vi "Turn off heating pins (SILAR).vi"(0 "Arduino Resource In":T1={"VISA resource"="", "Board Type"=enum."Uno", "Connection Type"=enum."USB / Serial", "Bytes Per Packet (15)"=15}, 5 "Error In":errorcluster) -> (14 "Arduino Resource Out":T1={"VISA resource"="", "Board Type"=enum."Uno", "Connection Type"=enum."USB / Serial", "Bytes Per Packet (15)"=15}, 19 "Error Out":errorcluster)   [LabVIEW 2012]
uses:
  <vilib>/LabVIEW Interface for Arduino/Type Defs/Arduino Resource.ctl
  <vilib>/LabVIEW Interface for Arduino/Type Defs/Board Type.ctl
  <vilib>/LabVIEW Interface for Arduino/LabVIEW Interface for Arduino.lvlib
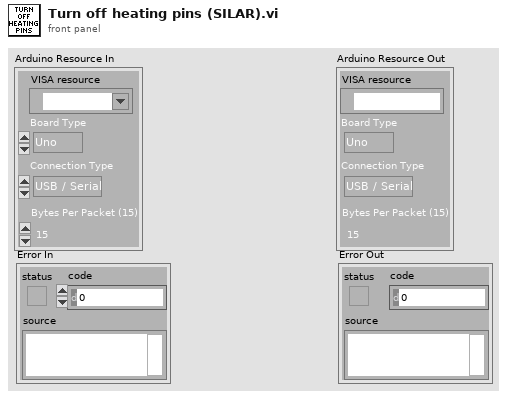
[diagram p1: front panel]
types:
  T1 = typedef "LabVIEW Interface for Arduino.lvlib/Arduino Resource.ctl" = cluster{"VISA resource":refnum<visa-resource-name>, "Board Type":T2, "Connection Type":enum8{"USB / Serial"}, "Bytes Per Packet (15)":u8}
  T2 = typedef "LabVIEW Interface for Arduino.lvlib/Board Type.ctl" = enum16{"Uno", "Dimuelanove w/Atmega 328", "Mega 2560"}
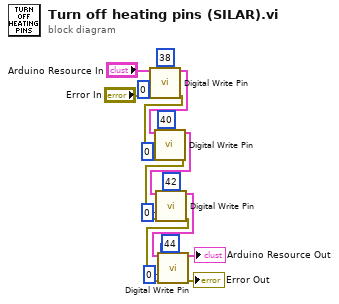
[diagram p0: block diagram]
diagram:
  n1 = call <vilib>:"Digital Write Pin.vi"("Arduino Resource"="Arduino Resource In", "Digital I/O Pin (0)"=u8 38, "Value (0)"=u8 0, "error in"="Error In") -> ("Arduino Resource"=w15:T1, "error out"=w16:errorcluster)  [unwired: 10 in]
  n2 = call <vilib>:"Digital Write Pin.vi"("Arduino Resource"=w15, "Digital I/O Pin (0)"=u8 40, "Value (0)"=u8 0, "error in"=w16) -> ("Arduino Resource"=w9:T1, "error out"=w10:errorcluster)  [unwired: 10 in]
  n3 = call <vilib>:"Digital Write Pin.vi"("Arduino Resource"=w9, "Digital I/O Pin (0)"=u8 42, "Value (0)"=u8 0, "error in"=w10) -> ("Arduino Resource"=w11:T1, "error out"=w12:errorcluster)  [unwired: 10 in]
  n4 = call <vilib>:"Digital Write Pin.vi"("Arduino Resource"=w11, "Digital I/O Pin (0)"=u8 44, "Value (0)"=u8 0, "error in"=w12) -> ("Arduino Resource"=→"Arduino Resource Out":T1, "error out"=→"Error Out":errorcluster)  [unwired: 10 in]
